vi "Get Type.vi"(8 "error in (no error)":errorcluster, 11 "LED Array in":refnum<class "LED Array.lvclass">) -> (0 "error out":errorcluster, 2 "Item Type":T1, 3 "LED Array out":refnum<class "LED Array.lvclass">)   [LabVIEW 2020, in "LED Array.lvclass"]
uses:
  LED Array.lvclass
  Item/Item Type.ctl
  Item/Item.lvclass
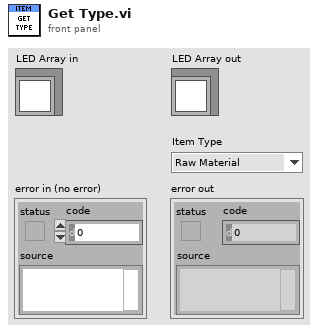
[diagram p1: front panel]
types:
  T1 = typedef "Item.lvclass/Item Type.ctl" = enum16{"Raw Material", "Component", "Module", "Product"}
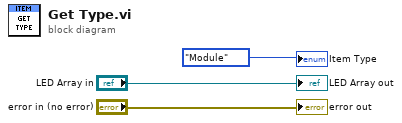
[diagram p0: block diagram]
diagram:
  "error out" <- "error in (no error)"
  "LED Array out" <- "LED Array in"
  "Item Type" <- Item_Type."Module" ("Item Type")
